vi "DOE Testing Quality Check.vi"(0 "Cold Water Temp Input":dbl, 1 "Hot Water Temp Input":dbl, 2 "Cold Water Pressure Input":dbl, 3 "Hot Water Pressure Input":dbl, 5 "Error In":errorcluster) -> (14 "Cold Water Temp Avg":dbl, 15 "Hot Water Temp Avg":dbl, 16 "Cold Water Pressure Avg":dbl, 17 "Hot Water Pressure Avg":dbl, 19 "Error Out":errorcluster)   [LabVIEW 2019]
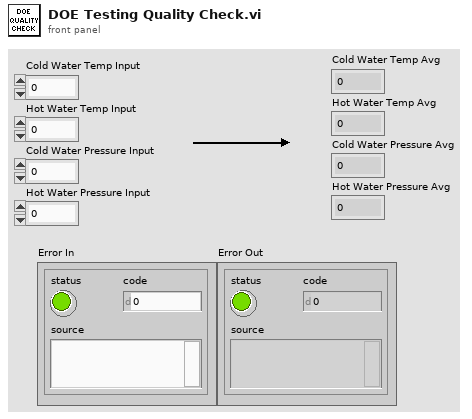
[diagram p1: front panel]
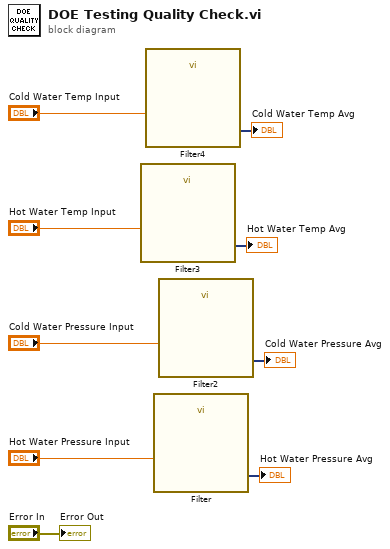
[diagram p0: block diagram]
diagram:
  n1 = call "Filter3"("Signal"="Hot Water Temp Input") -> ("Filtered Signal"=→"Hot Water Temp Avg":dynamicdata)  [unwired: 9 in, 1 out]
  n2 = call "Filter4"("Signal"="Cold Water Temp Input") -> ("Filtered Signal"=→"Cold Water Temp Avg":dynamicdata)  [unwired: 9 in, 1 out]
  n3 = call "Filter"("Signal"="Hot Water Pressure Input") -> ("Filtered Signal"=→"Hot Water Pressure Avg":dynamicdata)  [unwired: 9 in, 1 out]
  n4 = call "Filter2"("Signal"="Cold Water Pressure Input") -> ("Filtered Signal"=→"Cold Water Pressure Avg":dynamicdata)  [unwired: 9 in, 1 out]
  "Error Out" <- "Error In"
